vi "Clean Up Actor.vi"(8 "error in (no error)":errorcluster, 11 "Car Wash Console in":refnum<class "Car Wash Display.lvclass">) -> (0 "error out":errorcluster, 3 "Car Wash Console out":refnum<class "Car Wash Display.lvclass">)   [LabVIEW 2016, in "CLD Exam - Car Wash.lvlib" / "Car Wash Display.lvclass"]
doc: "--\nCopyright © 2017 Composed SystemsI All rights reserved.\n\nAuthor: Jon McBee <jon.mcbee@composed.io>\n\nThis library is provided \"AS IS\" ,WITHOUT WARRANTIES OR\nCONDITIONS OF ANY KIND, either express or implied.\n\nComposed Systems -- composed.io\n\nStream 0.0.1.1\nJon McBee - Composed Systems\nCopyright (c) 2017, Composed Systems"
uses:
  Car Wash Display.lvclass
  D:/Repos/Stream/software/Mediator/Classes/Mediated Actor/Mediated Actor.lvclass
  Mediator/Classes/Message Broker Interface/Message Broker Interface.lvclass
  Mediator/Classes/Mediated Synchronous Actor/Mediated Synchronous Actor.lvclass
  Mediator/Classes/Mediated Actor/Mediated Actor.lvclass
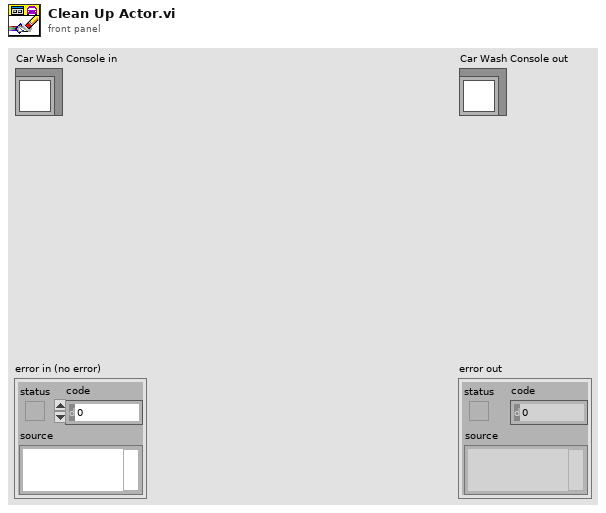
[diagram p1: front panel]
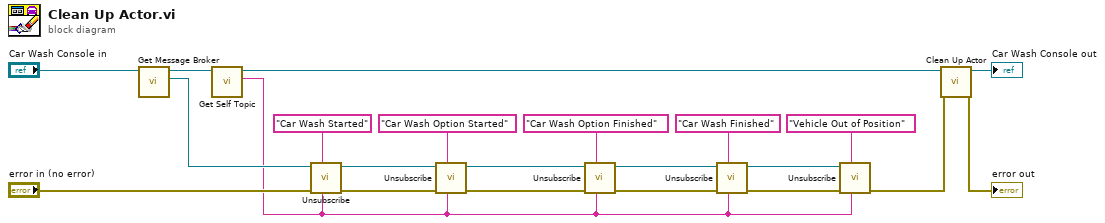
[diagram p0: block diagram]
diagram:
  n1 = call "Get Message Broker.vi"("Mediated Actor in"="Car Wash Console in") -> ("Message Broker"=w19:refnum<class "Message Broker Interface.lvclass">, "Mediated Actor out"=w20:refnum<class "Car Wash Display.lvclass">)  [unwired: 9 in]
  n2 = call "Get Self Topic.vi"("Mediated Actor in"=w20) -> ("Topic.Self"=w2:string, "Mediated Actor out"=w16:refnum<class "Car Wash Display.lvclass">)  [unwired: 9 in]
  n3 = call-dynamic "Unsubscribe.vi"("Subscriber Name"=w2, "Topic Name"="Car Wash Started", "error in (no error)"="error in (no error)", "Message Broker Interface in"=w19) -> ("error out"=w12:errorcluster, "Message Broker Interface out"=w13:refnum<class "Message Broker Interface.lvclass">)  [unwired: 6 in]
  n4 = call-dynamic "Unsubscribe.vi"("Subscriber Name"=w2, "Topic Name"="Car Wash Option Started", "error in (no error)"=w12, "Message Broker Interface in"=w13) -> ("error out"=w6:errorcluster, "Message Broker Interface out"=w7:refnum<class "Message Broker Interface.lvclass">)  [unwired: 6 in]
  n5 = call-dynamic "Unsubscribe.vi"("Subscriber Name"=w2, "Topic Name"="Car Wash Option Finished", "error in (no error)"=w6, "Message Broker Interface in"=w7) -> ("error out"=w11:errorcluster, "Message Broker Interface out"=w10:refnum<class "Message Broker Interface.lvclass">)  [unwired: 6 in]
  n6 = call-dynamic "Unsubscribe.vi"("Subscriber Name"=w2, "Topic Name"="Car Wash Finished", "error in (no error)"=w11, "Message Broker Interface in"=w10) -> ("error out"=w3:errorcluster, "Message Broker Interface out"=w4:refnum<class "Message Broker Interface.lvclass">)  [unwired: 6 in]
  n7 = call-dynamic "Unsubscribe.vi"("Subscriber Name"=w2, "Topic Name"="Vehicle Out of Position", "error in (no error)"=w3, "Message Broker Interface in"=w4) -> ("error out"=w1:errorcluster)  [unwired: 6 in, 1 out]
  n8 = call-parent "Clean Up Actor.vi"("error in (no error)"=w1, "Mediated Actor in"=w16) -> ("error out"=→"error out":errorcluster, "Mediated Actor out"=→"Car Wash Console out":refnum<class "Car Wash Display.lvclass">)  [unwired: 8 in]
